vi "VI-Move and Connect Ref Array.vi"(2 "Components":T1, 11 "error in (no error)":errorcluster) -> (15 "error out":errorcluster)   [LabVIEW 2015]
uses:
  VI-Reg Event Components.ctl
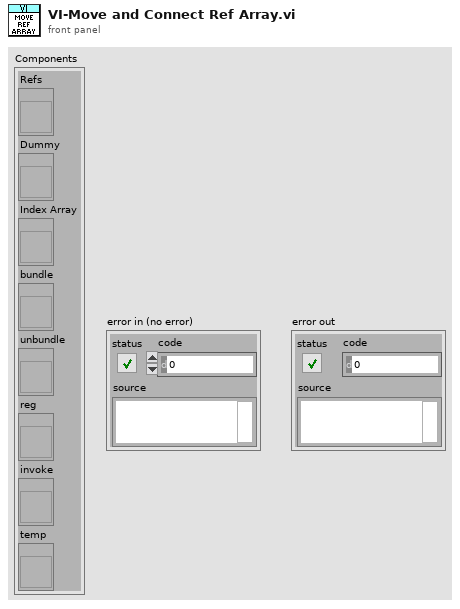
[diagram p1: front panel]
types:
  T1 = typedef "VI-Reg Event Components.ctl" = cluster{"Refs":refnum<vi>, "Dummy":refnum<vi>, "Index Array":refnum<vi>, "bundle":refnum<vi>, "unbundle":refnum<vi>, "reg":refnum<vi>, "invoke":refnum<vi>, "temp":refnum<vi>}
  T2 = typedef "LVPositionTypeDef.ctl" = cluster{"Left":i32, "Top":i32}
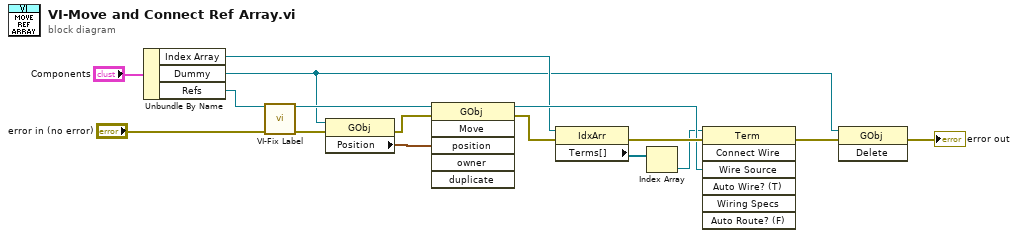
[diagram p0: block diagram]
diagram:
  n1 = Unbundle By Name("Components") -> ("Index Array"=w4:refnum<vi>, "Dummy"=w2:refnum<vi>, "Refs"=w5:refnum<vi>)
  n2 = call "VI-Fix Label.vi"("GObject in"=w5, "error in (no error)"="error in (no error)") -> ("GObject out"=w8:refnum<vi>, "error out"=w10:errorcluster)  [unwired: 12 in]
  n3 = property class="GObj"(reference=w2, error in=w10) -> (error out=w11:errorcluster, "Position"=w9:T2)  [unwired: 1 out]
  n4 = invoke class="GObj" method="Move"(reference=w8, error in=w11, "position"=w9) -> (reference out=w15:refnum<vi>, error out=w12:errorcluster)  [unwired: 3 in, 4 out]
  n5 = property class="IdxArr"(reference=w4, error in=w12) -> (error out=w16:errorcluster, "Terms[]"=w13:refnum<vi>[])  [unwired: 1 out]
  n6 = Index Array(array=w13) -> (element=w14:refnum<vi>)  [unwired: 1 in]
  n7 = invoke class="Term" method="Connect Wire"(reference=w14, error in=w16, "Wire Source"=w15) -> (error out=w3:errorcluster)  [unwired: 4 in, 6 out]
  n8 = invoke class="GObj" method="Delete"(reference=w2, error in=w3) -> (error out=→"error out":errorcluster)  [unwired: 1 in, 2 out]
